vi "io-find-by-tag.vi"(10 "Tag":string, 11 "IOConfigs in":T1[](array[typedef]) {"calibration"."Y" format="%#.3f"; "calibration"."X" format="%#.3f"; "ADDR" format="%04d"}) -> (3 "Filtered IOConfigs out":T1[](array[typedef]) {"calibration"."Y" format="%#.3f"; "calibration"."X" format="%#.3f"; "ADDR" format="%04d"})   [LabVIEW 2024]
uses:
  controls/IONode.ctl
  controls/type.address.ctl
  controls/enum.io.type.ctl
  controls/enum.io.mode.ctl
  controls/typeXyPoint.ctl
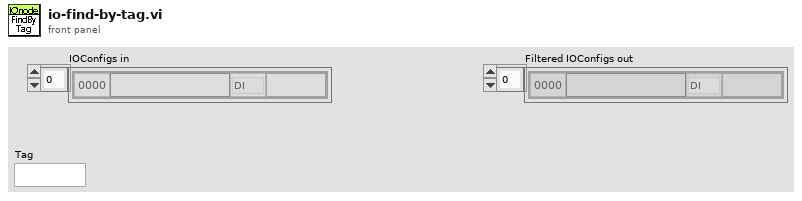
[diagram p1: front panel]
types:
  T1 = typedef "IONode.ctl" = cluster{"ADDR":T2, "Label":string, "Type":T3, "Mode":T4, "Value":string, "Tags":string, "calibration":T5[]}
  T2 = typedef "type.address.ctl" = u16
  T3 = typedef "enum.io.type.ctl" = enum16{"Type", "DI", "DO", "AI", "AO", "VL", "BUF"}
  T4 = typedef "enum.io.mode.ctl" = enum16{"Mode", "RIO", "SIM"}
  T5 = typedef "typeXyPoint.ctl" = cluster{"X":dbl, "Y":dbl}
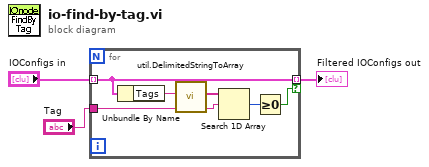
[diagram p0: block diagram]
diagram:
  n1 = for {
    tunnel: "Tag" -> [w7]
    tunnel: "IOConfigs in" -> [w6] mode=indexing
    tunnel: [w6] -> w2 mode=indexing if=w4
    n2 = Unbundle By Name(w6) -> ("Tags"=w9:string)
    n3 = call "util.DelimitedStringToArray.vi"("delimitaed string"=w9) -> ("array out"=w8:string[])  [unwired: 10 in]
    n4 = Search 1D Array(1D array=w8, element=w7) -> (index of element=w5:i32)  [unwired: 1 in]
    n5 = Greater Or Equal To 0?(x=w5) -> (x >= 0?=w4:bool)
  }
  "Filtered IOConfigs out" <- w2
